vi "Actor Core.vi"(8 "error in":errorcluster, 11 "Measurement_Binary in":refnum<class "Measurement_Binary.lvclass">) -> (0 "error out":errorcluster, 3 "Actor out":refnum<class "Actor.lvclass">)   [LabVIEW 2020, in "Measurement_Binary.lvlib" / "Measurement_Binary.lvclass"]
doc: "(<B>Filename</B>: Actor Framework.lvlib:Actor.lvclass:Actor Core.vi)\n\nReceives messages to the actor, reacts to them, and initiates any error handling that may shut the actor down.\n\nDescendant classes may override this VI to append parallel tasks for the actor to complete while it handles messages. Overrides use the Call Parent Class Method node."
uses:
  Measurement_Binary.lvclass
  C:/Program Files/National Instruments/LabVIEW 2020/vi.lib/ActorFramework/Actor/Actor.lvclass
  <vilib>/ActorFramework/Actor/Actor.lvclass
  <vilib>/ActorFramework/Actor/Actor.lvclass/Actor.ctl
  Measurement_Binary.lvclass/Measurement_Binary.ctl
  Binary counter Messages/Graph Data Msg/Graph Data Msg.lvclass/Graph Data Msg.ctl
  <vilib>/ActorFramework/Message Enqueuer/Message Enqueuer.lvclass/Message Enqueuer.ctl
  <vilib>/ActorFramework/Message Enqueuer/Enqueue.vi
  Binary counter Messages/Graph Data Msg/Graph Data Msg.lvclass
  C:/Program Files/National Instruments/LabVIEW 2020/vi.lib/ActorFramework/Message/Message.lvclass
  <vilib>/ActorFramework/Message Priority Queue/Priority Enqueue.vi
panel:
  out "Boolean":bool[](array[boolean])
  out "Start/stop":bool
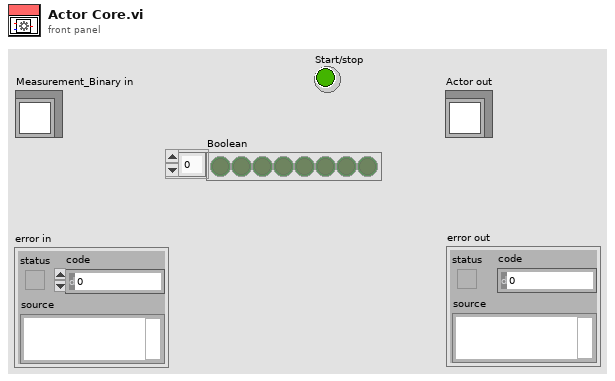
[diagram p1: front panel]
types:
  T1 = cluster{"Start/stop":refnum<user-event>, "Exit":refnum<user-event>, "Minimo":refnum<user-event>, "Maximo":refnum<user-event>}
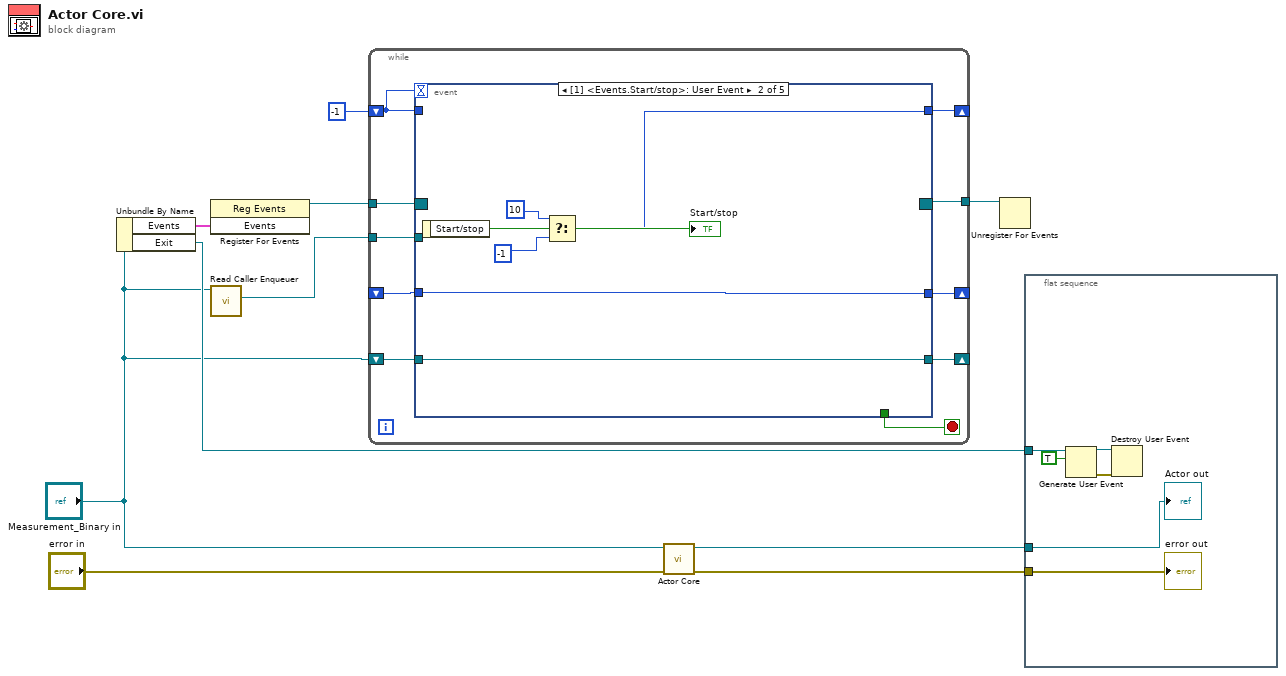
[diagram p0: block diagram]
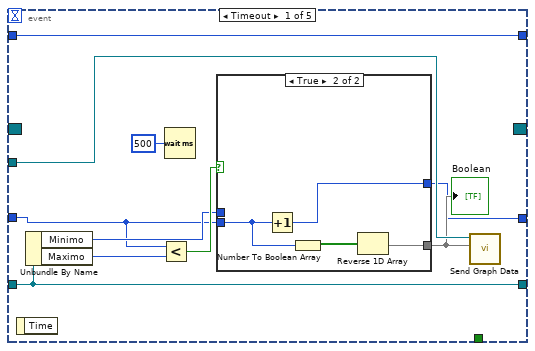
[diagram p2: hidden frame]
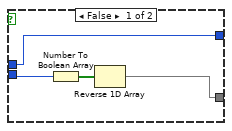
[diagram p3: hidden frame]
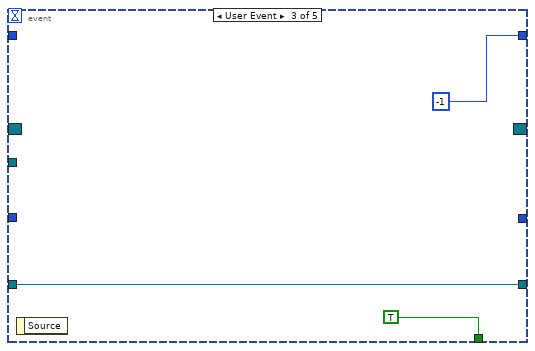
[diagram p4: hidden frame]
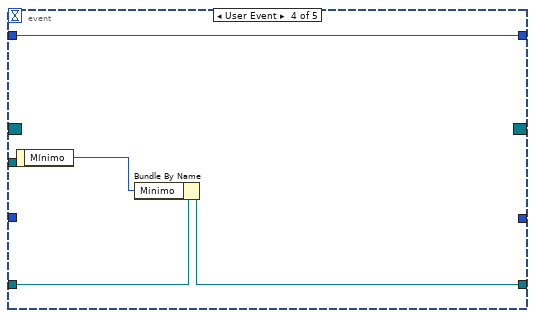
[diagram p5: hidden frame]
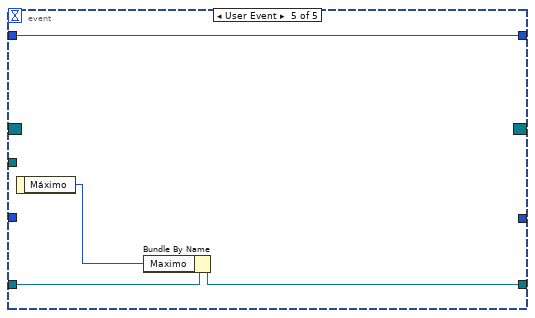
[diagram p6: hidden frame]
diagram:
  n1 = Unbundle By Name("Measurement_Binary in") -> ("Events"=w7:T1, "Exit"=w2:refnum<user-event>)
  n2 = register-events(w7) -> (reference out=w6:refnum<event-registration>)  [unwired: 2 in, 1 out]
  n3 = call <vilib>:"Read Caller Enqueuer.vi"("Actor"="Measurement_Binary in") -> ("Caller Enqueuer"=w3:refnum<class "Message Enqueuer.lvclass">)  [unwired: 10 in]
  n4 = while {
    tunnel: w6 -> [w20]
    shift-right: [w18] -> _
    shift-left: -1 -> [w19]
    tunnel: [w17] -> w4
    shift-right: [w14] -> _
    shift-left: "Measurement_Binary in" -> [w15]
    tunnel: w3 -> [w13]
    shift-right: [w11] -> _
    shift-left: _ -> [w12]
    stop <- w16 stop-if-true
    n5 = event shown="[1] <Events.Start/stop>: User Event" {
      selector: w20 -> [_ _ _ _ _]
      dyn-events: [_ _ _ _ _] -> w17
      timeout: w19 -> [_ _ _ _ _]
      tunnel: w19 -> [w30 _ _ w48 w52]
      tunnel: [w30 w41 -1 ("t") w48 w52] -> w18
      tunnel: [_ _ TRUE _ _] -> w16
      tunnel: w15 -> [w29 w40 w45 w51 w55]
      tunnel: [w29 w40 w45 w50 w54] -> w14
      tunnel: w13 -> [w26 _ _ _ _]
      tunnel: w12 -> [w22 w39 _ _ _]
      tunnel: [w21 w39 _ _ _] -> w11
      event Timeout {
        n6 = event-data() -> ()  [unwired: 1 in, 1 out]
        n7 = Unbundle By Name(w29) -> ("Minimo"=w25:u8, "Maximo"=w28:u8)
        n8 = Less?(x=w22, y=w28) -> (x < y?=w27:bool)
        n9 = Wait (ms)(milliseconds to wait=u32 500) -> ()  [unwired: 1 out]
        n10 = case shown="True" w27 {
          tunnel: w22 -> [w34 w35]
          tunnel: [w31 w38] -> w21
          tunnel: [w32 w36] -> w24
          tunnel: w25 -> [w31 _]
          frame False {
            n11 = Number To Boolean Array(number=w34) -> (Boolean array=w33:bool[])
            n12 = Reverse 1D Array(array=w33) -> (reversed array=w32:bool[])
          }
          frame True {
            n13 = Increment(x=w35) -> (x+1=w38:u8)
            n14 = Number To Boolean Array(number=w35) -> (Boolean array=w37:bool[])
            n15 = Reverse 1D Array(array=w37) -> (reversed array=w36:bool[])
          }
        }
        "Boolean" <- w24
        n16 = call "Send Graph Data.vi"("Leds 2"=w24, "Message Enqueuer"=w26) -> ()  [unwired: 8 in, 2 out]
      }
      event User Event {
        n17 = event-data() -> ("Start/stop"=w44:bool)  [unwired: 1 in]
        "Start/stop" <- w44
        n18 = Select(t=10, s=w44, f=-1) -> (s? t:f=w41:i32)
      }
      event User Event {
        n19 = event-data() -> ()  [unwired: 1 in, 1 out]
      }
      event User Event {
        n20 = event-data() -> ("Mínimo"=w49:u8)  [unwired: 1 in]
        n21 = Bundle By Name(cluster=w51, "Minimo"=w49) -> (w50:refnum<class "Measurement_Binary.lvclass">)
      }
      event User Event {
        n22 = event-data() -> ("Máximo"=w53:u8)  [unwired: 1 in]
        n23 = Bundle By Name(cluster=w55, "Maximo"=w53) -> (w54:refnum<class "Measurement_Binary.lvclass">)
      }
    }
  }
  n24 = call-parent "Actor Core.vi"("error in"="error in", "Actor in"="Measurement_Binary in") -> ("error out"=w10:errorcluster, "Actor out"=w9:refnum<class "Actor.lvclass">)  [unwired: 8 in]
  n25 = Unregister For Events(event registration refnum=w4) -> ()  [unwired: 1 in, 1 out]
  n26 = flat-sequence {
    tunnel: w10 -> [w61]
    tunnel: w9 -> [w60]
    tunnel: w2 -> [w59]
    frame #0 {
      n27 = Generate User Event(user event=w59, event data cluster=TRUE ("event data")) -> (user event out=w56:refnum<user-event>, error out=w57:errorcluster)  [unwired: 2 in]
      n28 = Destroy User Event(user event=w56, error in=w57) -> ()  [unwired: 1 out]
      "error out" <- w61
      "Actor out" <- w60
    }
  }
